vi "Duplicate Routing Channel RTM.vi"(8 "error in (no error)":errorcluster, 11 "Node Ptr":u64 format="%.0x") -> (0 "error out":errorcluster)   [LabVIEW 2017, in "Routing and Faulting System Explorer.lvlib"]
uses:
  Routing and Faulting System Explorer.lvlib
  9b785d74-dca3-4762-b15d-51e0b6148e04.vi
  Scripting/Routing and Faulting Scripting.lvlib
  <vilib>/NI Veristand/Custom Device Tools/Custom Device Utility Library/Custom Device Utility Library.lvlib
  <vilib>/NI Veristand/Custom Device API/Custom Device API.lvlib
panel:
  in  "Tag":string
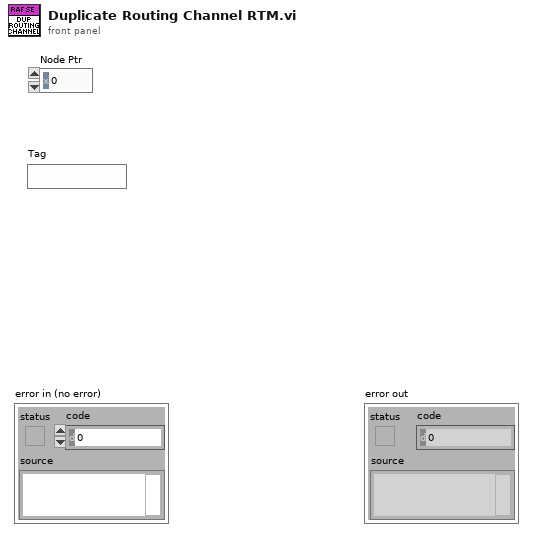
[diagram p1: front panel]
types:
  T1 = typedef "Routing and Faulting Shared.lvlib/Channel States.ctl" = T2[]
  T2 = typedef "Routing and Faulting Shared.lvlib/Routing State.ctl" = cluster{"Name":string, "Description":string, "Value":i32, "Connection List":T3[]}
  T3 = typedef "Routing and Faulting Shared.lvlib/Connection.ctl" = cluster{"Resource":string, "Source":string, "Destination":string}
  T4 = typedef "Custom Device API.lvlib/Custom Device Item Ref.ctl" = u64
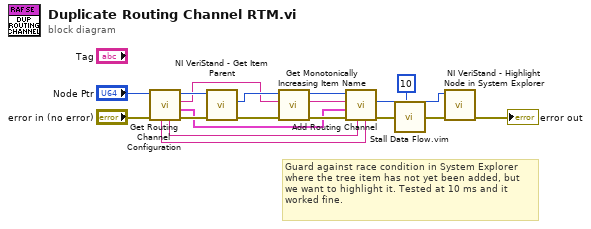
[diagram p0: block diagram]
diagram:
  # "Guard against race condition in System Explorer\nwhere the tree item has not yet been added, but\nwe want to highlight it. Tested at 10 ms and it\nworked fine."
  n1 = call "Get Routing Channel Configuration.vi"("error in (no error)"="error in (no error)", "Channel Ref in"="Node Ptr") -> ("error out"=w10:errorcluster, "State Configurations"=w5:T1, "Channel Name"=w7:string, "Channel Ref out"=w9:T4, "Initial State"=w4:string, "Description"=w3:string)  [unwired: 4 in]
  n2 = call <vilib>:"NI VeriStand - Get Item Parent.vi"("error in (no error)"=w10, "Item Ref in"=w9) -> ("error out"=w6:errorcluster, "Parent Ref"=w8:T4)  [unwired: 6 in, 2 out]
  n3 = call "Get Monotonically Increasing Item Name.vi"("error in (no error)"=w6, "Desired Name"=w7, "Section Ptr"=w8) -> ("error out"=w17:errorcluster, "New Item Name"=w16:string, "Section Ptr out"=w18:T4)  [unwired: 6 in]
  n4 = call "Add Routing Channel.vi"("Description"=w3, "Initial State"=w4, "error in (no error)"=w17, "State Configurations"=w5, "Channel Name"=w16, "Routing Channels Ref in"=w18) -> ("error out"=w15:errorcluster, "Channel Ref"=w13:T4)  [unwired: 3 in, 1 out]
  n5 = call "Stall Data Flow.vim"("value in"=w15, "milliseconds to wait"=u32 10) -> ("value out"=w2:errorcluster)  [unwired: 1 out]
  n6 = call <vilib>:"NI VeriStand - Highlight Node in System Explorer.vi"("error in (no error)"=w2, "Item Ref in"=w13) -> ("error out"=→"error out":errorcluster)  [unwired: 8 in, 1 out]
